vi "save.vi"(4 "OME parameters":T3, 6 "OME XMLElement":refnum<class "XMLElement.lvclass">, 7 "saving parameters":T1={"write OME header?"=TRUE, "save as list file?"=FALSE, "force format?"=enum."uint16", "multiplication factor"=1.0, "offset"=0.0}, 8 "error in (no error)":errorcluster, 10 "path":path, 11 "ImageCollection in":refnum<class "ImageCollection.lvclass">) -> (0 "error out":errorcluster, 3 "ImageCollection out":refnum<class "ImageCollection.lvclass">)   [LabVIEW 2010, in "ImageCollection.lvclass"]
uses:
  ImageCollection.lvclass
  OME_parameters_cluster.ctl
  dimension_order_enum.ctl
  XMLElement/XMLElement/XMLElement.lvclass
  saving_parameters_cluster.ctl
  Image/Image/target_format_enum.ctl
  Image/Image/Image.lvclass
  libraries/TIFFManagement/TIFFManagement.lvlib
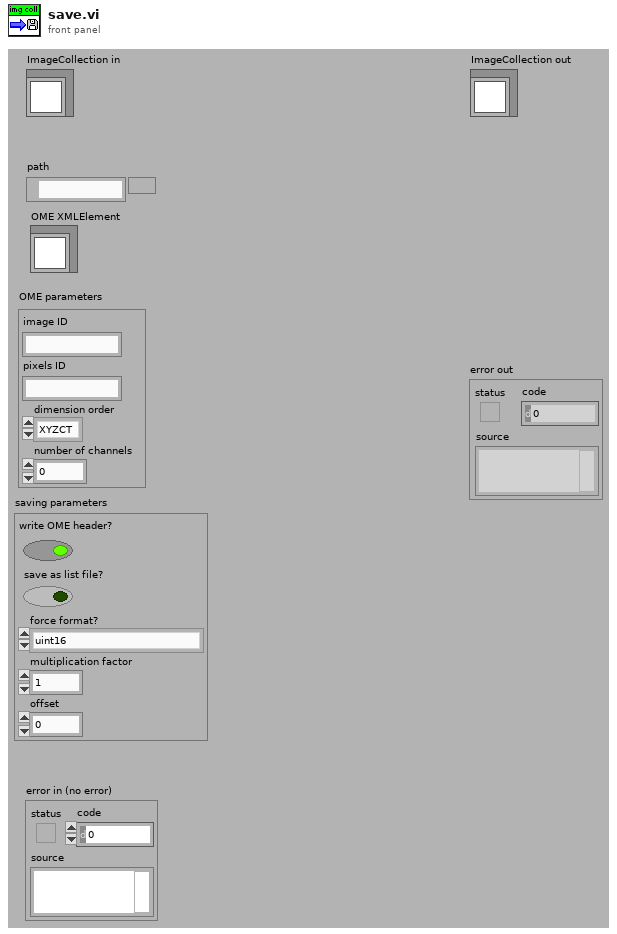
[diagram p1: front panel]
types:
  T1 = typedef "ImageCollection.lvclass/saving_parameters_cluster.ctl" = cluster{"write OME header?":bool, "save as list file?":bool, "force format?":T2, "multiplication factor":dbl, "offset":dbl}
  T2 = typedef "target_format_enum.ctl" = enum16{"don't force", "uint8", "uint16", "int16", "uint32", "int32", "single float"}
  T3 = typedef "OME_parameters_cluster.ctl" = cluster{"image ID":string, "pixels ID":string, "dimension order":T4, "number of channels":i32}
  T4 = typedef "dimension_order_enum.ctl" = enum16{"XYZCT", "XYZTC", "XYCTZ", "XYCZT", "XYTCZ", "XYTZC"}
  T5 = enum16{"open", "replace", "create", "open or create", "replace or create", "replace or create with confirmation"}
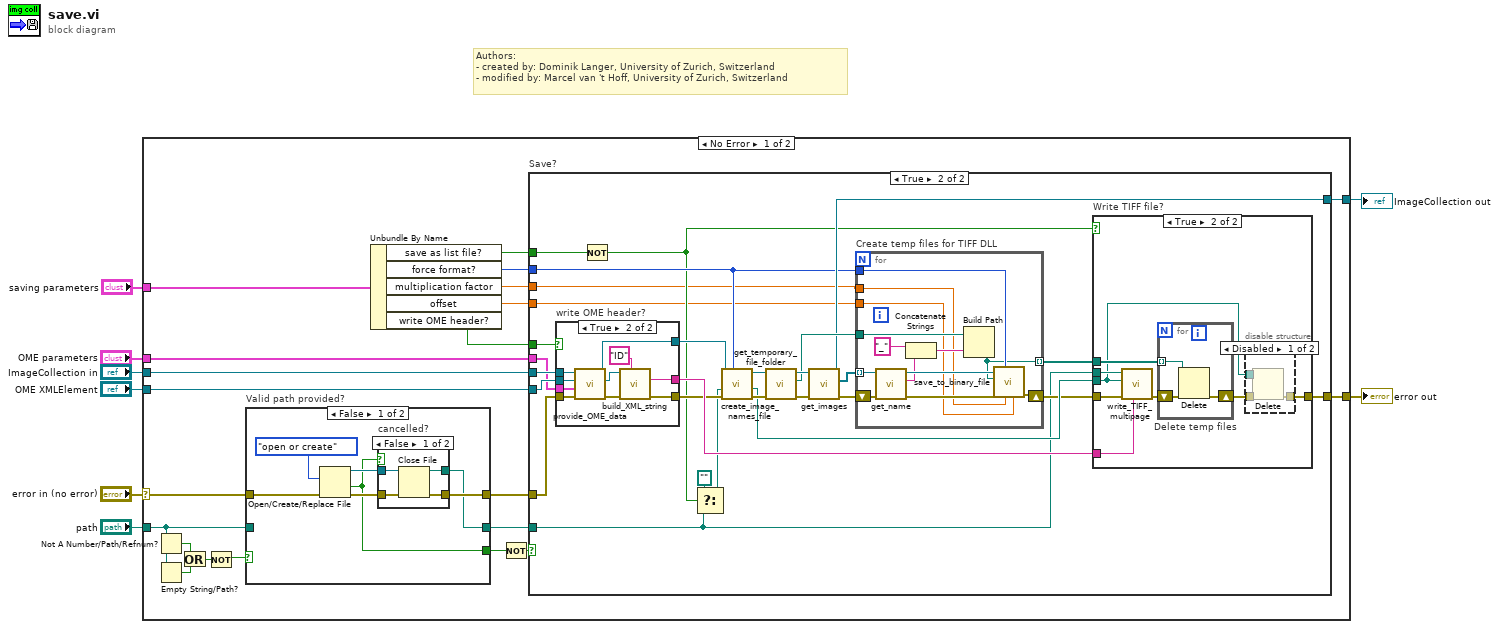
[diagram p0: block diagram]
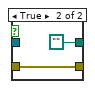
[diagram p6: hidden frame]
diagram:
  # "Authors: \n- created by: Dominik Langer, University of Zurich, Switzerland\n- modified by: Marcel van 't Hoff, University of Zurich, Switzerland"
  n1 = case shown="No Error" "error in (no error)" {
    selector: "error in (no error)" -> [w24 w117]
    tunnel: [w27 w117] -> w8
    tunnel: [w28 w116] -> w6
    tunnel: "ImageCollection in" -> [w29 w116]
    tunnel: "path" -> [w21 _]
    tunnel: "OME XMLElement" -> [w15 _]
    tunnel: "OME parameters" -> [w16 _]
    tunnel: "saving parameters" -> [w14 _]
    frame No Error {
      n2 = Not A Number/Path/Refnum?(number/path/refnum=w21) -> (NaN/Path/Refnum?=w25:bool)
      n3 = Empty String/Path?(string/path=w21) -> (empty?=w26:bool)
      n4 = Or(x=w25, y=w26) -> (x .or. y?=w20:bool)
      n5 = Not(x=w20) -> (.not. x?=w19:bool)
      n6 = case "Valid path provided?" shown="False" w19 {
        tunnel: w24 -> [w104 w115]
        tunnel: [w103 w115] -> w23
        tunnel: [w101 w114] -> w22
        tunnel: w21 -> [_ w114]
        tunnel: [w102 _] -> w17
        frame False {
          n7 = Open/Create/Replace File(error in=w104, operation (0:open)=T5."open or create") -> (refnum out=w105:refnum<file>, cancelled=w102:bool, error out=w106:errorcluster)  [unwired: 4 in]
          n8 = case "cancelled?" shown="False" w102 {
            tunnel: w105 -> [w111 _]
            tunnel: w106 -> [w110 w112]
            tunnel: [w109 w112] -> w103
            tunnel: [w108 path ""] -> w101
            frame False {
              n9 = Close File(refnum=w111, error in=w110) -> (path=w108:path, error out=w109:errorcluster)
            }
            frame True {
            }
          }
        }
        frame True {
        }
      }
      n10 = Unbundle By Name(w14) -> ("save as list file?"=w13:bool, "force format?"=w12:T2, "multiplication factor"=w11:dbl, "offset"=w10:dbl, "write OME header?"=w9:bool)
      n11 = Not(x=w17) -> (.not. x?=w18:bool)
      n12 = case "Save?" shown="True" w18 {
        tunnel: w29 -> [w31 w58]
        tunnel: [w31 w45] -> w28
        tunnel: [w30 w44] -> w27
        tunnel: w23 -> [w30 w59]
        tunnel: w22 -> [_ w34]
        tunnel: w12 -> [_ w42]
        tunnel: w15 -> [_ w57]
        tunnel: w16 -> [_ w56]
        tunnel: w9 -> [_ w39]
        tunnel: w13 -> [_ w38]
        tunnel: w11 -> [_ w32]
        tunnel: w10 -> [_ w33]
        frame False {
        }
        frame True {
          n13 = case "write OME header?" shown="True" w39 {
            tunnel: w59 -> [w60 w71]
            tunnel: w58 -> [w61 w70]
            tunnel: w57 -> [_ w69]
            tunnel: w56 -> [_ w67]
            tunnel: [_ w65] -> w55
            tunnel: [w61 w64] -> w54
            tunnel: [w60 w62] -> w40
            frame False {
            }
            frame True {
              n14 = call "provide_OME_data.vi"("error in (no error)"=w71, "parameters"=w67, "OME XMLElement in"=w69, "ImageCollection in"=w70) -> ("error out"=w63:errorcluster, "OME XMLElement out"=w66:refnum<class "XMLElement.lvclass">, "ImageCollection out"=w64:refnum<class "ImageCollection.lvclass">)  [unwired: 5 in]
              n15 = call "build_XML_string.vi"("ID tag"="ID" ("id parameter name"), "error in (no error)"=w63, "Element in"=w66) -> ("error out"=w62:errorcluster, "string"=w65:string)  [unwired: 6 in, 1 out]
            }
          }
          n16 = Not(x=w38) -> (.not. x?=w37:bool)
          n17 = Select(t=path "", s=w37, f=w34) -> (s? t:f=w35:path)
          n18 = call "create_image_names_file.vi"("force format?"=w42, "error in (no error)"=w40, "file path in (can be empty)"=w35, "ImageCollection in"=w54) -> ("error out"=w51:errorcluster, "file path out"=w43:path, "ImageCollection out"=w50:refnum<class "ImageCollection.lvclass">)  [unwired: 1 in, 4 out]
          n19 = call-dynamic "get_temporary_file_folder.vi"("error in (no error)"=w51, "ImageCollection.lvclass in"=w50) -> ("error out"=w49:errorcluster, "temporary file folder"=w47:path, "ImageCollection.lvclass out"=w48:refnum<class "ImageCollection.lvclass">)  [unwired: 7 out]
          n20 = call-dynamic "get_images.vi"("error in (no error)"=w49, "ImageCollection.lvclass in"=w48) -> ("error out"=w53:errorcluster, "images"=w52:refnum<class "Image.lvclass">[], "ImageCollection.lvclass out"=w45:refnum<class "ImageCollection.lvclass">)  [unwired: 7 in]
          n21 = for "Create temp files for TIFF DLL" {
            shift-right: [w99] -> w41
            shift-left: w53 -> [w98]
            tunnel: w52 -> [w97] mode=indexing
            tunnel: w42 -> [w100]
            tunnel: w47 -> [w95]
            tunnel: [w93] -> w46 mode=indexing
            tunnel: w33 -> [w88]
            tunnel: w32 -> [w89]
            n22 = call-dynamic "get_name.vi"("error in (no error)"=w98, "Image in"=w97) -> ("error out"=w96:errorcluster, "name"=w92:string, "Image out"=w94:refnum<class "Image.lvclass">)  [unwired: 7 in]
            n23 = Concatenate Strings("_" ("string"), w92) -> (w90:string)
            n24 = Build Path(base path=w95, name or relative path=w90) -> (appended path=w93:path)
            n25 = call-dynamic "save_to_binary_file.vi"("offset (0)"=w88, "multiplication factor (1)"=w89, "force format?"=w100, "error in (no error)"=w96, "Path"=w93, "Image in"=w94) -> ("error out"=w99:errorcluster)  [unwired: 4 in, 1 out]
          }
          n26 = case "Write TIFF file?" shown="True" w37 {
            tunnel: w34 -> [_ w80]
            tunnel: w55 -> [_ w79]
            tunnel: w46 -> [_ w78]
            tunnel: [w72 w76] -> w44
            tunnel: w43 -> [_ w75]
            tunnel: w41 -> [w72 w74]
            frame False {
            }
            frame True {
              n27 = call "write_TIFF_multipage.vi"("description tag"=w79, "error in (no error)"=w74, "description file"=w75, "path in"=w80) -> ("error out"=w73:errorcluster)  [unwired: 6 in, 1 out]
              n28 = for "Delete temp files" {
                shift-right: [w86] -> w77
                shift-left: w73 -> [w87]
                tunnel: w78 -> [w85] mode=indexing
                n29 = Delete(path (use dialog)=w85, error in=w87) -> (error out=w86:errorcluster)  [unwired: 3 in, 2 out]
              }
              n30 = disable-structure shown="Disabled" {
                disable-tunnel: w77 -> [w83 w84]
                disable-tunnel: [w82 w84] -> w76
                disable-tunnel: w75 -> [w81 _]
                frame Disabled {
                  n31 = Delete(path (use dialog)=w81, error in=w83) -> (error out=w82:errorcluster)  [unwired: 3 in, 2 out]
                }
                frame Enabled {
                }
              }
            }
          }
        }
      }
    }
    frame Error {
    }
  }
  "error out" <- w8
  "ImageCollection out" <- w6
